vi "Write Description.vi"(10 "Description":string, 11 "Assertion Result In":refnum<class "Assertion Result.lvclass">) -> (3 "Assertion Result Out":refnum<class "Assertion Result.lvclass">)   [LabVIEW 2020, in "Assertion Result.lvclass"]
uses:
  Assertion Result.lvclass
  Assertion Result.lvclass/Assertion Result.ctl
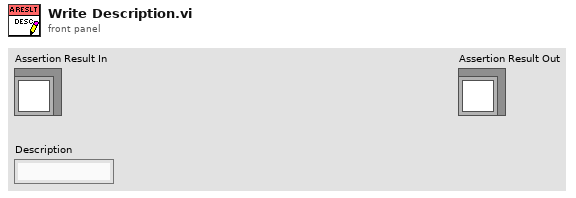
[diagram p1: front panel]
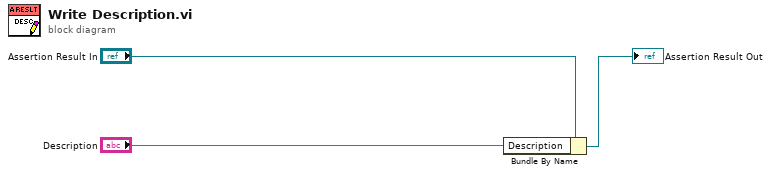
[diagram p0: block diagram]
diagram:
  n1 = Bundle By Name(cluster="Assertion Result In", "Description"="Description") -> (→"Assertion Result Out":refnum<class "Assertion Result.lvclass">)
